vi "dataframes_DTU.vi"(9 "input cluster":T1 {"payload" format="%x"; "timestamp" format="%<%.7X\n%x>T"; "type" items=["CAN Data"=0, "CAN Remote"=1, "CAN Bus Error"=2, "CAN 2.0 Data"=8, "CAN FD Data"=16, "CAN FD+BRS Data"=24, "J1939 Data"=192, "Delay"=224, "Log Trigger"=225, "Start Trigger"=226]; "identifier" format="%x"}, 10 "frame data":T1[](array[typedef]) {"payload" format="%x"; "timestamp" format="%<%.7X\n%x>T"; "type" items=["CAN Data"=0, "CAN Remote"=1, "CAN Bus Error"=2, "CAN 2.0 Data"=8, "CAN FD Data"=16, "CAN FD+BRS Data"=24, "J1939 Data"=192, "Delay"=224, "Log Trigger"=225, "Start Trigger"=226]; "identifier" format="%x"}) -> (2 "frame data 2":T1[](array[typedef]) {"payload" format="%x"; "timestamp" format="%<%.7X\n%x>T"; "type" items=["CAN Data"=0, "CAN Remote"=1, "CAN Bus Error"=2, "CAN 2.0 Data"=8, "CAN FD Data"=16, "CAN FD+BRS Data"=24, "J1939 Data"=192, "Delay"=224, "Log Trigger"=225, "Start Trigger"=226]; "identifier" format="%x"})   [LabVIEW 2024]
uses:
  <vilib>/xnet/xnet.llb/XNET Frame CAN.ctl
  <vilib>/xnet/xnet.llb/XNET Frame Type CAN.ctl
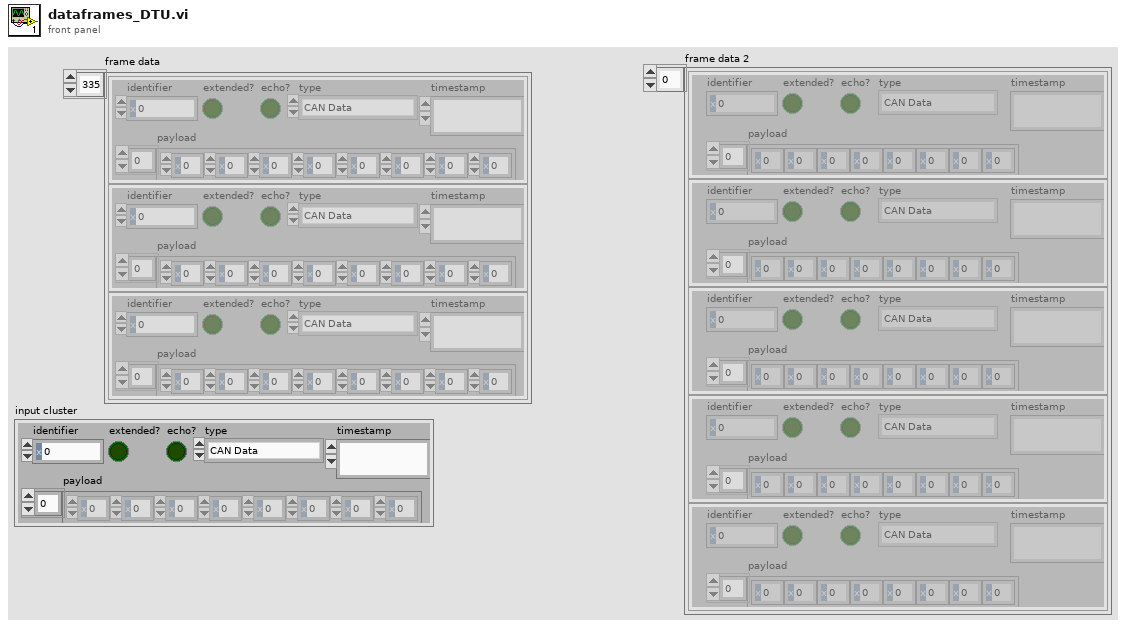
[diagram p1: front panel]
types:
  T1 = typedef "XNET Frame CAN.ctl" = cluster{"timestamp":timestamp, "payload":u8[], "identifier":u32, "type":T2, "extended?":bool, "echo?":bool}
  T2 = typedef "XNET Frame Type CAN.ctl" = u8
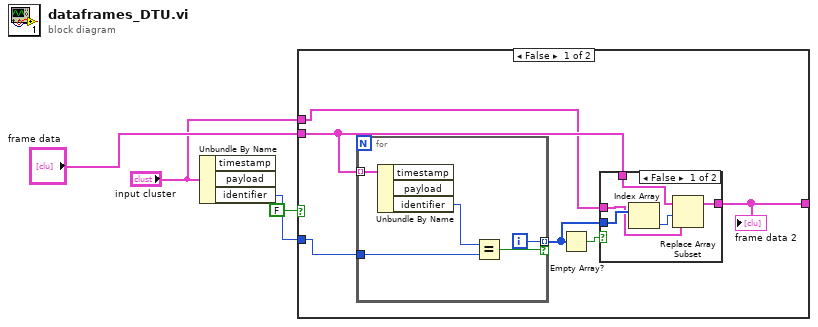
[diagram p0: block diagram]
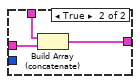
[diagram p2: hidden frame]
diagram:
  n1 = Unbundle By Name("input cluster") -> ("identifier"=w2:u32)  [unwired: 2 out]
  n2 = case shown="False" FALSE {
    tunnel: [w10 w24] -> _
    tunnel: "frame data" -> [w6 w24]
    tunnel: w2 -> [w7 _]
    tunnel: "input cluster" -> [w5 _]
    frame False {
      n3 = for {
        tunnel: [w15] -> w9 mode=indexing if=w14
        tunnel: w6 -> [w13] mode=indexing
        tunnel: w7 -> [w11]
        i -> [w15]
        n4 = Unbundle By Name(w13) -> ("identifier"=w12:u32)  [unwired: 2 out]
        n5 = Equal?(x=w12, y=w11) -> (x = y?=w14:bool)
      }
      n6 = Empty Array?(array=w9) -> (empty?=w8:bool)
      n7 = case shown="False" w8 {
        tunnel: [w18 w23] -> w10
        tunnel: w9 -> [w20 _]
        tunnel: w6 -> [w17 w22]
        tunnel: w5 -> [w16 w21]
        frame False {
          n8 = Index Array(array=w20) -> (element=w19:i32)  [unwired: 1 in]
          n9 = Replace Array Subset(array=w17, new element=w16, index=w19) -> (w18:T1[])
        }
        frame True {
          n10 = Build Array (concatenate)(w22, w21) -> (w23:T1[])
        }
      }
      "frame data 2" <- w10
    }
    frame True {
    }
  }
